vi "issue_timestep_response.vi"(2 "timestep (in)":dbl, 5 "error in (no error)":errorcluster) -> (19 "error out":errorcluster)   [LabVIEW 2016]
uses:
  support/controls/queue_assistant_actions.ctl
  support/controls/entity.ctl
  support/controls/entity_type.ctl
  support/controls/group.ctl
  support/controls/response.ctl
  support/controls/response_type.ctl
  support/controls/queue_type.ctl
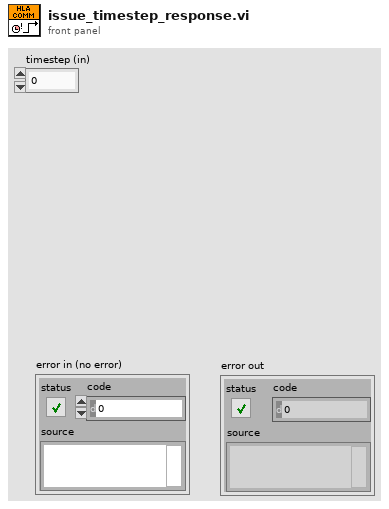
[diagram p1: front panel]
types:
  T1 = typedef "entity.ctl" = cluster{"type":T2, "classPath":string, "params":string[][], "instanceName":string}
  T2 = typedef "entity_type.ctl" = string
  T3 = typedef "queue_assistant_actions.ctl" = enum16{"--- unused ---", "bulk_enq_ahead", "bulk_enq_behind", "destroy", "empty?", "enq_ahead", "enq_behind", "flush", "get_queues", "init"}
  T4 = typedef "queue_type.ctl" = enum16{"all", "dostep", "entities_incoming", "entities_outoing", "response"}
  T5 = typedef "response_type.ctl" = string
  T6 = typedef "response.ctl" = cluster{"respType":T5, "flattenedContent":string}
  T7 = typedef "group.ctl" = cluster{"timeStep":dbl, "entities":T1[]}
  T8 = typedef "queue_references.ctl" = cluster{"entities_in":refnum<queue>, "entities_out":refnum<queue>, "timestep":refnum<queue>, "response":refnum<queue>}
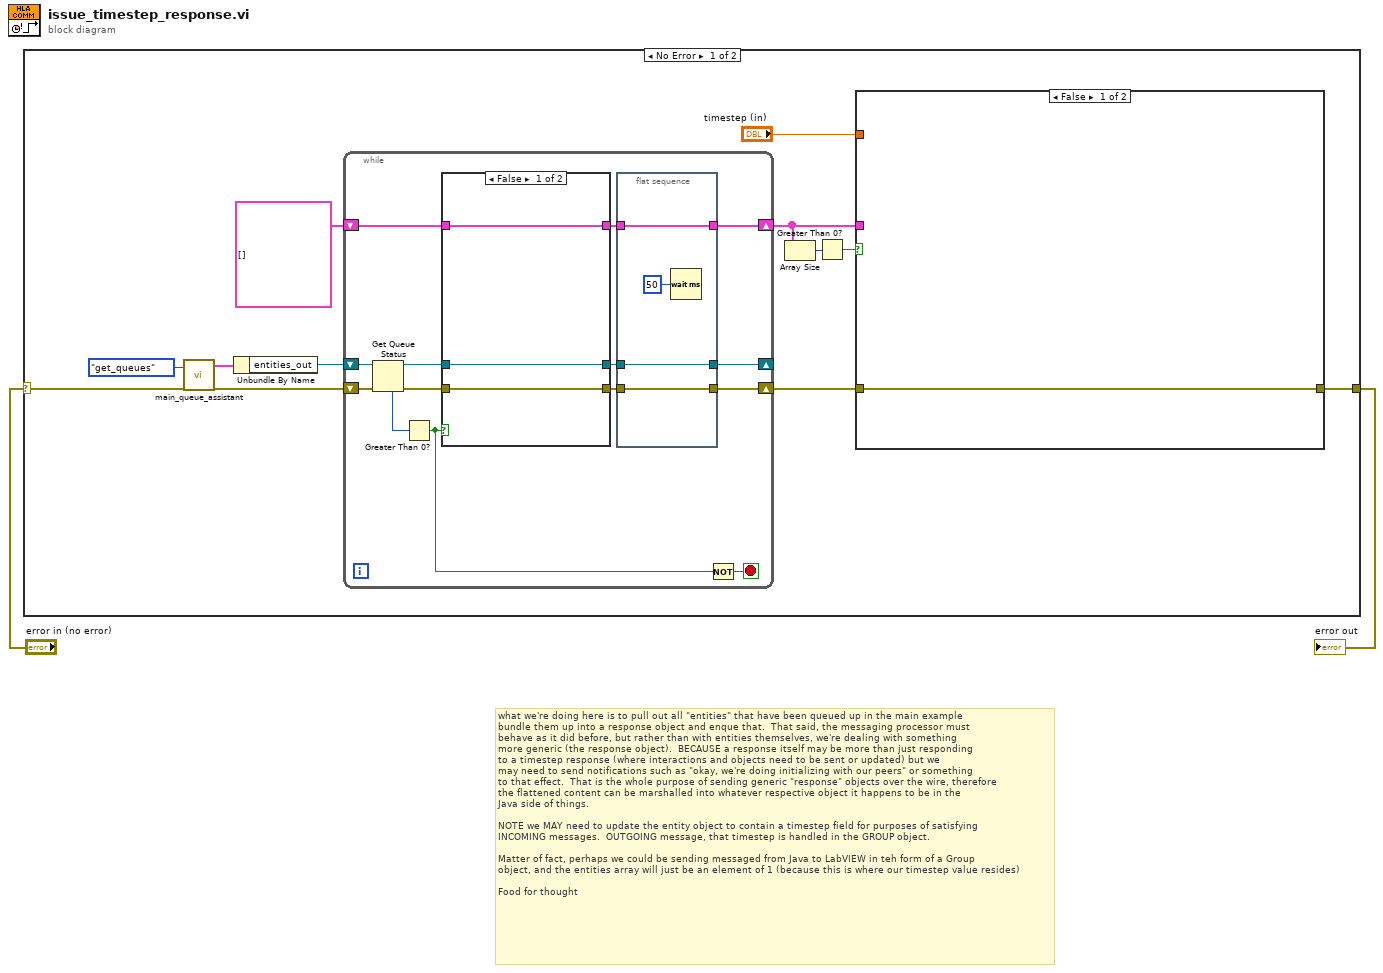
[diagram p0: block diagram]
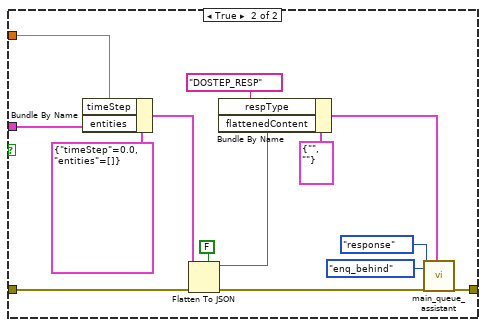
[diagram p2: hidden frame]
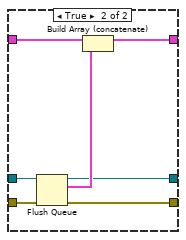
[diagram p3: hidden frame]
diagram:
  # "what we're doing here is to pull out all \"entities\" that have been queued up in the main example\nbundle them up into a response object and enque that.  That said, the messaging processor must\nbehave as it did before, but rather than with entities themselves, we're dealing with something\nmore generic (the response object).  BECAUSE a response itself may be more than just responding\nto a timestep response (where interactions and objects need to be sent or updated) but we \nmay need to send notifications such as \"okay, we're doing initializing with our peers\" or something\nto that effect.  That is the whole purpose of sending generic \"response\" objects over the wire, therefore\nthe flattened content can be marshalled into whatever respective object it happens to be in the\nJava side of things.\n\nNOTE we MAY need to update the entity object to contain a timestep field for purposes of satisfying\nINCOMING messages.  OUTGOING message, that timestep is handled in the GROUP object.\n\nMatter of fact, perhaps we could be sending messaged from Java to LabVIEW in teh form of a Group\nobject, and the entities array will just be an element of 1 (because this is where our timestep value resides)\n\nFood for thought"
  n1 = case shown="No Error" "error in (no error)" {
    selector: "error in (no error)" -> [w4 w58]
    tunnel: [w3 w58] -> w1
    frame No Error {
      n2 = call "main_queue_assistant.vi"("action (enq_behind = def)"=queue_assistant_actions."get_queues", "error in (no error)"=w4) -> ("refs (out)"=w13:T8, "error out"=w11:errorcluster)  [unwired: 15 in, 1 out]
      n3 = Unbundle By Name(w13) -> ("entities_out"=w12:refnum<queue>)
      n4 = while {
        shift-right: [w32] -> w7
        shift-left: T1[] [] ("remaining elements") -> [w38]
        shift-right: [w31] -> _
        shift-left: w12 -> [w43]
        shift-right: [w30] -> w8
        shift-left: w11 -> [w42]
        stop <- w36 stop-if-true
        n5 = Get Queue Status(queue=w43, error in (no error)=w42) -> (queue out=w40:refnum<queue>, error out=w39:errorcluster, # elements in queue=w41:i32)  [unwired: 1 in, 5 out]
        n6 = Greater Than 0?(x=w41) -> (x > 0?=w37:bool)
        n7 = case shown="False" w37 {
          tunnel: w40 -> [w49 w57]
          tunnel: w39 -> [w48 w56]
          tunnel: w38 -> [w50 w55]
          tunnel: [w49 w53] -> w34
          tunnel: [w48 w52] -> w33
          tunnel: [w50 w51] -> w35
          frame False {
          }
          frame True {
            n8 = Flush Queue(queue=w57, error in (no error)=w56) -> (queue out=w53:refnum<queue>, remaining elements=w54:T1[], error out=w52:errorcluster)
            n9 = Build Array (concatenate)(w55, w54) -> (w51:T1[])
          }
        }
        n10 = flat-sequence {
          tunnel: [w47] -> w32
          tunnel: w35 -> [w47]
          tunnel: [w46] -> w31
          tunnel: w34 -> [w46]
          tunnel: [w45] -> w30
          tunnel: w33 -> [w45]
          frame #0 {
            n11 = Wait (ms)(milliseconds to wait=u32 50) -> ()  [unwired: 1 out]
          }
        }
        n12 = Not(x=w37) -> (.not. x?=w36:bool)
      }
      n13 = Array Size(array=w7) -> (size(s)=w6:i32)
      n14 = Greater Than 0?(x=w6) -> (x > 0?=w5:bool)
      n15 = case shown="False" w5 {
        tunnel: "timestep (in)" -> [_ w28]
        tunnel: w8 -> [w15 w26]
        tunnel: w7 -> [_ w17]
        tunnel: [w15 w16] -> w3
        frame False {
        }
        frame True {
          n16 = Bundle By Name(cluster=T7 {"timeStep"=0.0, "entities"=[]} ("group"), "timeStep"=w28, "entities"=w17) -> (w25:T7)
          n17 = Flatten To JSON(enable LabVIEW extensions? (T)=FALSE, anything=w25, error in (no error)=w26) -> (JSON string=w23:string, 11:w19:errorcluster)
          n18 = Bundle By Name(cluster=T6 {"respType"="", "flattenedContent"=""} ("response"), "respType"=T5 "DOSTEP_RESP", "flattenedContent"=w23) -> (w18:T6)
          n19 = call "main_queue_assistant.vi"("queue_type (def=all)"=queue_type."response", "action (enq_behind = def)"=queue_assistant_actions."enq_behind", "error in (no error)"=w19, "response"=w18) -> ("error out"=w16:errorcluster)  [unwired: 13 in, 2 out]
        }
      }
    }
    frame Error {
    }
  }
  "error out" <- w1
